vi "UnconnectedTest.vi"() -> ()   [LabVIEW 2013]
panel:
  out "x-y":u32
  in  "Y Center / mm":dbl format="%#_13g"
  in  "X Center / mm":dbl format="%#_13g"
  out "Time":dbl
  in  "Precision":i32
  in  "Radius / mm":dbl format="%#_13g"
  in  "Shape":enum16{"Self-defined", "Circle"}(ring)=enum."Circle"
  out "x resolution":dbl
  out "y resolution":dbl
  out "X":i32
  out "Y":i32
  out "Case":i16
  out "XY Graph":cluster{dbl[], dbl[]}(graph)
  in  "Polygon Point":dbl[][](array[numeric])
  in  "Size input solution":enum16{"Dynamic Size", "Fixed Size"}(ring)=enum."Fixed Size"
  in  "Y move Maximum / mm":dbl
  in  "X move Maximum / mm":dbl
  in  "Y step / mm":dbl
  in  "X step / mm":dbl
  in  "Initial YPos / mm":dbl
  in  "Initial XPos / mm":dbl
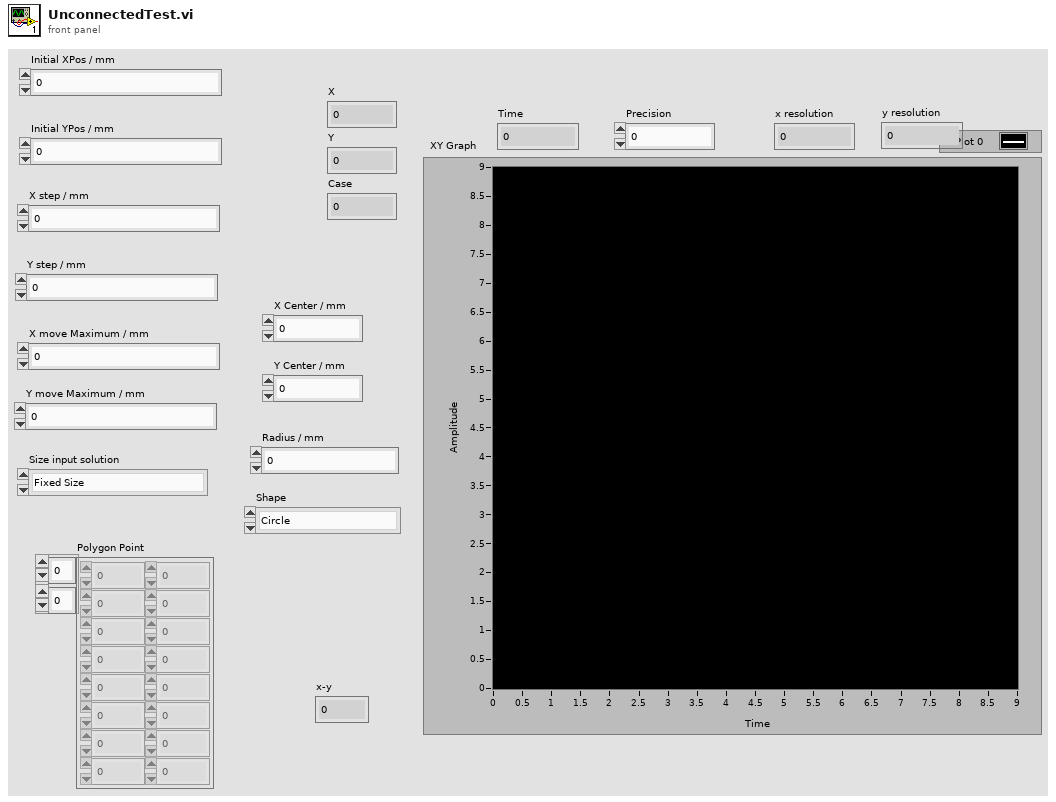
[diagram p1: front panel]
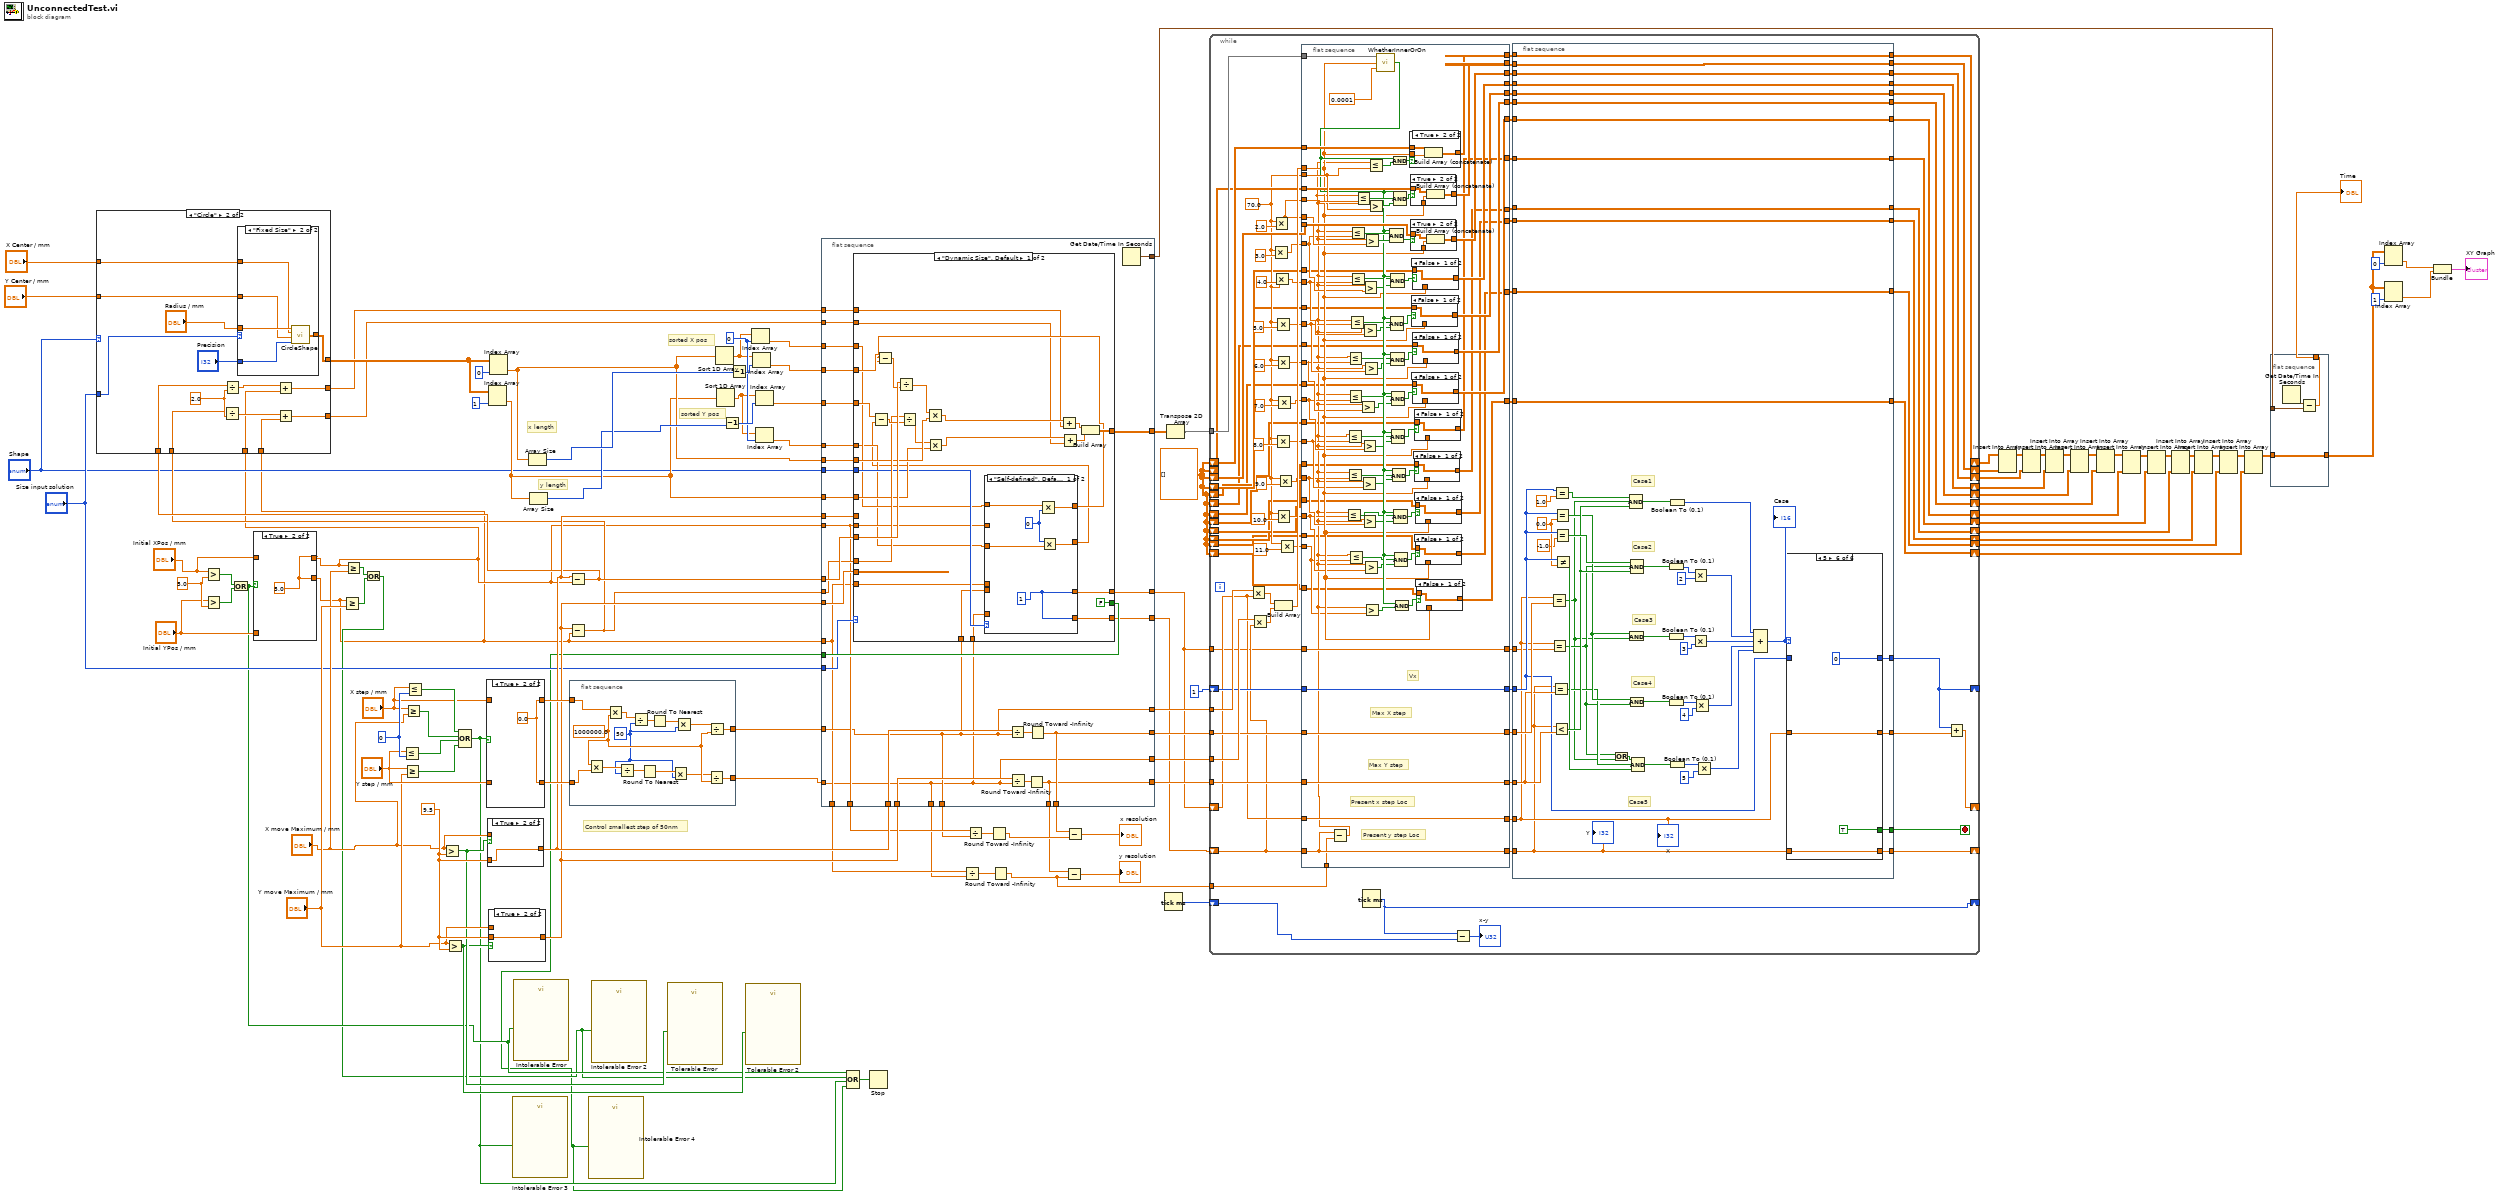
[diagram p0: block diagram]
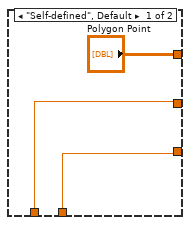
[diagram p2: hidden frame]
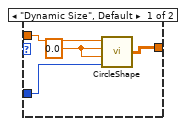
[diagram p3: hidden frame]
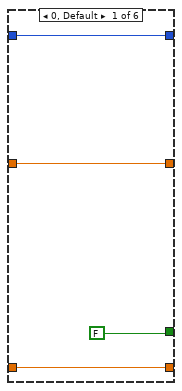
[diagram p4: hidden frame]
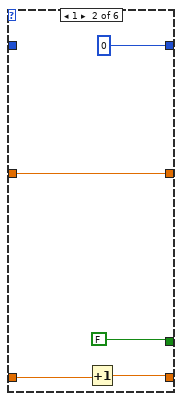
[diagram p5: hidden frame]
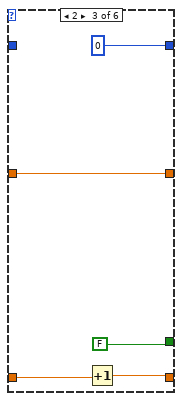
[diagram p6: hidden frame]
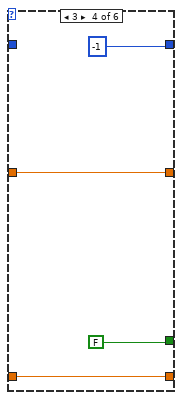
[diagram p7: hidden frame]
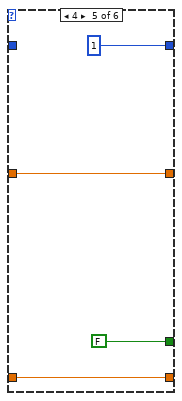
[diagram p8: hidden frame]
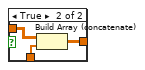
[diagram p9: hidden frame]
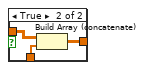
[diagram p10: hidden frame]
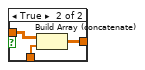
[diagram p11: hidden frame]
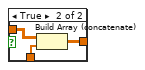
[diagram p12: hidden frame]
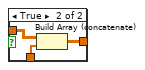
[diagram p13: hidden frame]
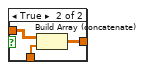
[diagram p14: hidden frame]
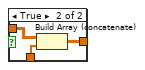
[diagram p15: hidden frame]
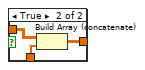
[diagram p16: hidden frame]
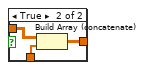
[diagram p17: hidden frame]
diagram:
  w57 = 0 ("index")
  w22 = dbl[][] []
  w104 = 0
  w105 = 9.5
  w110 = 5.0
  # "sorted Y pos"
  # "sorted X pos"
  # "Control smallest step of 50nm"
  # "y length"
  # "x length"
  n1 = Greater?(x="Initial XPos / mm", y=w110) -> (0:w109:bool)
  n2 = Greater?(x="Initial YPos / mm", y=w110) -> (0:w108:bool)
  n3 = Or(x=w109, y=w108) -> (x .or. y?=w64:bool)
  n4 = case shown="True" w64 {
    tunnel: "Initial XPos / mm" -> [w112 _]
    tunnel: "Initial YPos / mm" -> [w111 _]
    tunnel: [w112 w113] -> w45
    tunnel: [w111 w113] -> w44
    frame False {
    }
    frame True {
      w113 = 5.0
    }
  }
  n5 = Greater Or Equal?(x=w44, y="Y move Maximum / mm") -> (x >= y?=w92:bool)
  n6 = Greater Or Equal?(x=w45, y="X move Maximum / mm") -> (x >= y?=w93:bool)
  n7 = Or(x=w93, y=w92) -> (x .or. y?=w63:bool)
  n8 = Less Or Equal?(x="Y step / mm", y=w104) -> (x <= y?=w101:bool)
  n9 = Greater Or Equal?(x="Y step / mm", y="Y move Maximum / mm") -> (x >= y?=w100:bool)
  n10 = Greater Or Equal?(x="X step / mm", y="X move Maximum / mm") -> (x >= y?=w102:bool)
  n11 = Less Or Equal?(x="X step / mm", y=w104) -> (x <= y?=w103:bool)
  n12 = Greater?(x="X move Maximum / mm", y=w105) -> (0:w91:bool)
  n13 = Greater?(x="Y move Maximum / mm", y=w105) -> (0:w90:bool)
  n14 = Compound Arithmetic op=OR(w103, w102, w101, w100) -> (w62:bool)
  n15 = case shown="True" w62 {
    tunnel: "X step / mm" -> [w115 _]
    tunnel: "Y step / mm" -> [w114 _]
    tunnel: [w115 w116] -> w89
    tunnel: [w114 w116] -> w88
    frame False {
    }
    frame True {
      w116 = 0.0
    }
  }
  n16 = case shown="True" w91 {
    tunnel: w105 -> [_ w118]
    tunnel: "X move Maximum / mm" -> [w117 _]
    tunnel: [w117 w118] -> w77
    frame False {
    }
    frame True {
    }
  }
  n17 = case shown="True" w90 {
    tunnel: w105 -> [_ w120]
    tunnel: "Y move Maximum / mm" -> [w119 _]
    tunnel: [w119 w120] -> w76
    frame False {
    }
    frame True {
    }
  }
  n18 = call "Intolerable Error 3"("Enable"=w62) -> ()  [unwired: 9 in, 2 out]
  n19 = call "Intolerable Error"("Enable"=w64) -> ()  [unwired: 9 in, 2 out]
  n20 = Subtract(x=w77, y=w45) -> (x-y=w70:dbl)
  n21 = Subtract(x=w76, y=w44) -> (x-y=w69:dbl)
  n22 = case shown="\"Circle\"" "Shape" {
    tunnel: ["Polygon Point" w136] -> w79
    tunnel: "Size input solution" -> [_ w135]
    tunnel: w70 -> [_ w131]
    tunnel: w69 -> [_ w130]
    tunnel: w44 -> [w121 w129]
    tunnel: w45 -> [w122 w128]
    tunnel: [w122 w127] -> w68
    tunnel: [w121 w126] -> w67
    tunnel: "X Center / mm" -> [_ w125]
    tunnel: "Y Center / mm" -> [_ w124]
    frame "Self-defined", Default {
    }
    frame "Circle" {
      w134 = 2.0
      n23 = Divide(x=w130, y=w134) -> (x/y=w132:dbl)
      n24 = Divide(x=w131, y=w134) -> (x/y=w133:dbl)
      n25 = case shown="\"Fixed Size\"" w135 {
        tunnel: "Radius / mm" -> [w141 w147]
        tunnel: "Precision" -> [w140 w146]
        tunnel: [w142 w145] -> w136
        tunnel: w125 -> [_ w144]
        tunnel: w124 -> [_ w143]
        frame "Dynamic Size", Default {
          w139 = 0.0 ("X initial")
          n26 = call "CircleShape.vi"("Precision"=w140, "Y initial"=w139, "X initial"=w139, "Radius"=w141) -> ("Output Point"=w142:dbl[][])
        }
        frame "Fixed Size" {
          n27 = call "CircleShape.vi"("Precision"=w146, "Y initial"=w143, "X initial"=w144, "Radius"=w147) -> ("Output Point"=w145:dbl[][])
        }
      }
      n28 = Add(x=w133, y=w128) -> (x+y=w127:dbl)
      n29 = Add(x=w132, y=w129) -> (x+y=w126:dbl)
    }
  }
  n30 = Index Array(array=w79, index (col)=1 ("disabled index (col)")) -> (element=w47:dbl[])  [unwired: 1 in]
  n31 = Index Array(array=w79, index (col)=0 ("disabled index (col)")) -> (element=w48:dbl[])  [unwired: 1 in]
  n32 = Array Size(array=w48) -> (size(s)=w50:i32)
  n33 = Array Size(array=w47) -> (size(s)=w49:i32)
  n34 = flat-sequence {
    tunnel: w89 -> [w161]
    tunnel: w88 -> [w158]
    tunnel: [w154] -> w87
    tunnel: [w153] -> w86
    frame #0 {
      w150 = 50
      w155 = 1000000.0
      n35 = Multiply(x=w155, y=w158) -> (x*y=w157:dbl)
      n36 = Multiply(x=w161, y=w155) -> (x*y=w160:dbl)
      n37 = Divide(x=w157, y=w150) -> (x/y=w156:dbl)
      n38 = Divide(x=w160, y=w150) -> (x/y=w159:dbl)
      n39 = Round To Nearest(number=w156) -> (nearest integer value=w151:dbl)
      n40 = Round To Nearest(number=w159) -> (nearest integer value=w152:dbl)
      n41 = Multiply(x=w151, y=w150) -> (x*y=w149:dbl)
      n42 = Multiply(x=w152, y=w150) -> (x*y=w148:dbl)
      n43 = Divide(x=w149, y=w155) -> (x/y=w153:dbl)
      n44 = Divide(x=w148, y=w155) -> (x/y=w154:dbl)
    }
  }
  n45 = call "Intolerable Error 4"("Enable"=w61) -> ()  [unwired: 9 in, 2 out]
  n46 = call "Intolerable Error 2"("Enable"=w63) -> ()  [unwired: 9 in, 2 out]
  n47 = call "Tolerable Error"("Enable"=w91) -> ()  [unwired: 9 in, 2 out]
  n48 = Sort 1D Array(array=w48) -> (sorted array=w55:dbl[])
  n49 = Sort 1D Array(array=w47) -> (sorted array=w56:dbl[])
  n50 = Decrement(x=w49) -> (x-1=w58:i32)
  n51 = Decrement(x=w50) -> (x-1=w59:i32)
  n52 = call "Tolerable Error 2"("Enable"=w90) -> ()  [unwired: 9 in, 2 out]
  n53 = Index Array(array=w55, index=w57) -> (element=w54:dbl)
  n54 = Index Array(array=w55, index=w59) -> (element=w53:dbl)
  n55 = Index Array(array=w56, index=w58) -> (element=w52:dbl)
  n56 = Index Array(array=w56, index=w57) -> (element=w51:dbl)
  n57 = flat-sequence {
    tunnel: w70 -> [w184]
    tunnel: w69 -> [w183]
    tunnel: w77 -> [w190]
    tunnel: w45 -> [w167]
    tunnel: w76 -> [w189]
    tunnel: w44 -> [w163]
    tunnel: [w188] -> w61
    tunnel: w87 -> [w166]
    tunnel: w86 -> [w162]
    tunnel: [w187] -> w81
    tunnel: [w165] -> w85
    tunnel: [w164] -> w84
    tunnel: [w162] -> w83
    tunnel: [w166] -> w82
    tunnel: [w182] -> w78
    tunnel: w68 -> [w181]
    tunnel: w67 -> [w180]
    tunnel: w77 -> [w179]
    tunnel: w76 -> [w178]
    tunnel: [w177] -> w72
    tunnel: [w176] -> w73
    tunnel: "Size input solution" -> [w175]
    tunnel: w54 -> [w174]
    tunnel: w53 -> [w173]
    tunnel: w52 -> [w172]
    tunnel: w51 -> [w171]
    tunnel: w48 -> [w170]
    tunnel: w47 -> [w169]
    tunnel: "Shape" -> [w168]
    tunnel: [w167] -> w33
    tunnel: [w166] -> w32
    tunnel: [w165] -> w30
    tunnel: [w164] -> w26
    tunnel: [w163] -> w25
    tunnel: [w162] -> w24
    frame #0 {
      n58 = case shown="\"Dynamic Size\", Default" w175 {
        tunnel: w170 -> [w213 w241]
        tunnel: w169 -> [w212 w240]
        tunnel: w173 -> [w219 w256]
        tunnel: w174 -> [w198 w254]
        tunnel: w172 -> [w218 w252]
        tunnel: w171 -> [w196 w249]
        tunnel: w184 -> [w217 _]
        tunnel: w183 -> [w214 _]
        tunnel: [w199 w242] -> w187
        tunnel: w190 -> [_ w255]
        tunnel: w167 -> [w207 w253]
        tunnel: w189 -> [_ w251]
        tunnel: w163 -> [w206 w250]
        tunnel: [FALSE w243] -> w188
        tunnel: w181 -> [w191 _]
        tunnel: w180 -> [w192 _]
        tunnel: w166 -> [w205 _]
        tunnel: w162 -> [w204 _]
        tunnel: [w202 w239] -> w177
        tunnel: [w203 w239] -> w176
        tunnel: w168 -> [w208 _]
        frame "Dynamic Size", Default {
          n59 = case shown="\"Self-defined\", Default" w208 {
            tunnel: w207 -> [_ w236]
            tunnel: w206 -> [_ w235]
            tunnel: w205 -> [_ w234]
            tunnel: w204 -> [_ w233]
            tunnel: [w225 w232] -> w203
            tunnel: [w225 w231] -> w202
            tunnel: w198 -> [w224 w230]
            tunnel: [w221 w229] -> w197
            tunnel: w196 -> [w223 w228]
            tunnel: [w220 w226] -> w195
            frame "Self-defined", Default {
              w222 = 0
              w225 = 1
              n60 = Multiply(x=w224, y=w222) -> (x*y=w221:dbl)
              n61 = Multiply(x=w222, y=w223) -> (x*y=w220:dbl)
            }
            frame "Circle" {
              w227 = 1.0
              n62 = Divide(x=w235, y=w233) -> (x/y=w237:dbl)
              n63 = Divide(x=w236, y=w234) -> (x/y=w238:dbl)
              n64 = Multiply(x=w230, y=w227) -> (x*y=w229:dbl)
              n65 = Multiply(x=w227, y=w228) -> (x*y=w226:dbl)
              n66 = Round Toward -Infinity(1:w238) -> (0:w232:dbl)
              n67 = Round Toward -Infinity(1:w237) -> (0:w231:dbl)
            }
          }
          n68 = Subtract(x=w218, y=w195) -> (x-y=w215:dbl)
          n69 = Subtract(x=w219, y=w197) -> (x-y=w216:dbl)
          n70 = Divide(x=w217, y=w216) -> (x/y=w194:dbl)
          n71 = Divide(x=w214, y=w215) -> (x/y=w193:dbl)
          n72 = Multiply(x=w194, y=w213) -> (x*y=w210:dbl[])
          n73 = Multiply(x=w193, y=w212) -> (x*y=w209:dbl[])
          n74 = Add(x=w210, y=w191) -> (x+y=w201:dbl[])
          n75 = Add(x=w209, y=w192) -> (x+y=w200:dbl[])
          n76 = Build Array(w201, w200) -> (w199:dbl[][])
        }
        frame "Fixed Size" {
          w239 = 1
          n77 = Greater?(x=w256, y=w255) -> (0:w247:bool)
          n78 = Less?(x=w254, y=w253) -> (x < y?=w248:bool)
          n79 = Greater?(x=w252, y=w251) -> (0:w246:bool)
          n80 = Less?(x=w249, y=w250) -> (x < y?=w245:bool)
          n81 = Compound Arithmetic op=OR(w248, w247, w246, w245) -> (w244:bool)
          n82 = case shown="True" w244 {
            tunnel: [FALSE TRUE] -> w243
            frame False {
            }
            frame True {
            }
          }
          n83 = Build Array(w241, w240) -> (w242:dbl[][])
        }
      }
      n84 = Divide(x=w179, y=w166) -> (x/y=w186:dbl)
      n85 = Divide(x=w178, y=w162) -> (x/y=w185:dbl)
      n86 = Round Toward -Infinity(1:w185) -> (0:w164:dbl)
      n87 = Round Toward -Infinity(1:w186) -> (0:w165:dbl)
      n88 = Get Date/Time In Seconds() -> (seconds since 1Jan1904=w182:timestamp)
    }
  }
  n89 = Compound Arithmetic op=OR(w64, w63, w62, w61) -> (w60:bool)
  n90 = Stop(stop? (T)=w60) -> ()
  n91 = Divide(x=w25, y=w24) -> (x/y=w27:dbl)
  n92 = Divide(x=w33, y=w32) -> (x/y=w34:dbl)
  n93 = Round Toward -Infinity(1:w34) -> (0:w29:dbl)
  n94 = Round Toward -Infinity(1:w27) -> (0:w23:dbl)
  n95 = Subtract(x=w26, y=w23) -> (x-y=→"y resolution":dbl)
  n96 = Subtract(x=w30, y=w29) -> (x-y=→"x resolution":dbl)
  n97 = Tick Count (ms)() -> (millisecond timer value=w43:u32)
  n98 = Transpose 2D Array(2D array=w81) -> (transposed array=w80:dbl[][])
  n99 = while {
    tunnel: w85 -> [w331]
    tunnel: w84 -> [w329]
    tunnel: w80 -> [w337]
    tunnel: w83 -> [w341]
    tunnel: w82 -> [w342]
    shift-right: [w322] -> _
    shift-left: 1 -> [w333]
    shift-right: [w321] -> _
    shift-left: w73 -> [w327]
    shift-right: [w320] -> _
    shift-left: w72 -> [w325]
    shift-right: [w319] -> w36
    shift-left: w22 -> [w336]
    tunnel: w73 -> [w317]
    shift-right: [w315] -> _
    shift-left: w43 -> [w316]
    shift-right: [w311] -> w35
    shift-left: w22 -> [w310]
    tunnel: w23 -> [w309]
    shift-right: [w304] -> w16
    shift-left: w22 -> [w306]
    shift-right: [w283] -> w15
    shift-left: w22 -> [w285]
    shift-right: [w280] -> w14
    shift-left: w22 -> [w282]
    shift-right: [w277] -> w13
    shift-left: w22 -> [w279]
    shift-right: [w274] -> w12
    shift-left: w22 -> [w276]
    shift-right: [w271] -> w10
    shift-left: w22 -> [w273]
    shift-right: [w268] -> w8
    shift-left: w22 -> [w270]
    shift-right: [w265] -> w7
    shift-left: w22 -> [w267]
    shift-right: [w262] -> w5
    shift-left: w22 -> [w264]
    shift-right: [w259] -> w2
    shift-left: w22 -> [w261]
    stop <- w324 stop-if-true
    w293 = 70.0
    n100 = Multiply(x=w342, y=w327) -> (x*y=w340:dbl)
    n101 = Multiply(x=w341, y=w325) -> (x*y=w339:dbl)
    n102 = Multiply(x=w293, y=3.0) -> (x*y=w303:dbl)
    n103 = Multiply(x=w293, y=2.0) -> (x*y=w308:dbl)
    n104 = Multiply(x=w293, y=4.0) -> (x*y=w299:dbl)
    n105 = Multiply(x=w293, y=5.0) -> (x*y=w292:dbl)
    n106 = Multiply(x=w293, y=8.0) -> (x*y=w289:dbl)
    n107 = Multiply(x=w293, y=6.0) -> (x*y=w291:dbl)
    n108 = Multiply(x=w293, y=10.0) -> (x*y=w287:dbl)
    n109 = Build Array(w340, w339) -> (w338:dbl[])
    n110 = Multiply(x=w293, y=7.0) -> (x*y=w290:dbl)
    n111 = Multiply(x=w293, y=9.0) -> (x*y=w288:dbl)
    n112 = Multiply(x=w293, y=11.0) -> (x*y=w286:dbl)
    n113 = flat-sequence {
      tunnel: w338 -> [w451]
      tunnel: w337 -> [w498]
      tunnel: w336 -> [w488]
      tunnel: [w503] -> w335
      tunnel: [w502] -> w334
      tunnel: w333 -> [w502]
      tunnel: [w501] -> w332
      tunnel: w331 -> [w501]
      tunnel: [w500] -> w330
      tunnel: w329 -> [w500]
      tunnel: [w499] -> w328
      tunnel: w327 -> [w499]
      tunnel: [w485] -> w326
      tunnel: w325 -> [w485]
      tunnel: [w496] -> w318
      tunnel: w317 -> [w496]
      tunnel: w293 -> [w489]
      tunnel: w308 -> [w490]
      tunnel: [w487] -> w312
      tunnel: w310 -> [w486]
      tunnel: w309 -> [w484]
      tunnel: w308 -> [w478]
      tunnel: w306 -> [w480]
      tunnel: [w479] -> w305
      tunnel: w303 -> [w450]
      tunnel: w299 -> [w448]
      tunnel: w292 -> [w447]
      tunnel: w291 -> [w446]
      tunnel: w290 -> [w445]
      tunnel: w289 -> [w444]
      tunnel: w288 -> [w443]
      tunnel: w287 -> [w442]
      tunnel: w286 -> [w440]
      tunnel: w285 -> [w439]
      tunnel: [w438] -> w284
      tunnel: w282 -> [w437]
      tunnel: [w436] -> w281
      tunnel: w279 -> [w435]
      tunnel: [w434] -> w278
      tunnel: w276 -> [w433]
      tunnel: [w432] -> w275
      tunnel: w273 -> [w431]
      tunnel: [w430] -> w272
      tunnel: w270 -> [w429]
      tunnel: [w428] -> w269
      tunnel: w267 -> [w427]
      tunnel: [w426] -> w266
      tunnel: w264 -> [w425]
      tunnel: [w424] -> w263
      tunnel: w261 -> [w423]
      tunnel: [w422] -> w260
      frame #0 {
        # "Max X step"
        # "Max Y step"
        # "Present y step Loc"
        # "Present x step Loc"
        # "Vx"
        n114 = Subtract(x=w485, y=w484) -> (x-y=w441:dbl)
        n115 = Less Or Equal?(x=w441, y=w442) -> (x <= y?=w455:bool)
        n116 = Less Or Equal?(x=w441, y=w444) -> (x <= y?=w459:bool)
        n117 = Less Or Equal?(x=w441, y=w443) -> (x <= y?=w457:bool)
        n118 = Less Or Equal?(x=w441, y=w446) -> (x <= y?=w463:bool)
        n119 = Less Or Equal?(x=w441, y=w445) -> (x <= y?=w461:bool)
        n120 = Less Or Equal?(x=w441, y=w440) -> (x <= y?=w453:bool)
        n121 = Less Or Equal?(x=w441, y=w447) -> (x <= y?=w465:bool)
        n122 = Less Or Equal?(x=w441, y=w450) -> (x <= y?=w482:bool)
        n123 = Less Or Equal?(x=w441, y=w448) -> (x <= y?=w467:bool)
        n124 = Less Or Equal?(x=w441, y=w490) -> (x <= y?=w492:bool)
        n125 = Greater?(x=w441, y=w446) -> (0:w460:bool)
        n126 = Greater?(x=w441, y=w444) -> (0:w456:bool)
        n127 = Greater?(x=w441, y=w445) -> (0:w458:bool)
        n128 = Greater?(x=w441, y=w443) -> (0:w454:bool)
        n129 = Greater?(x=w441, y=w448) -> (0:w464:bool)
        n130 = Greater?(x=w441, y=w450) -> (0:w466:bool)
        n131 = Greater?(x=w441, y=w447) -> (0:w462:bool)
        n132 = Greater?(x=w441, y=w442) -> (0:w452:bool)
        n133 = Greater?(x=w441, y=w478) -> (0:w481:bool)
        n134 = Greater?(x=w441, y=w440) -> (0:w449:bool)
        n135 = Less Or Equal?(x=w441, y=w489) -> (x <= y?=w494:bool)
        n136 = Greater?(x=w441, y=w489) -> (0:w491:bool)
        n137 = call "WhetherInnerOrOn.vi"("Error permitted"=0.0001, "JudgePoint"=w451, "InputPolygon"=w498) -> ("Point on or inside?"=w468:bool)
        n138 = Compound Arithmetic op=AND(w468, w482, w481) -> (w483:bool)
        n139 = Compound Arithmetic op=AND(w468, w465, w464) -> (w476:bool)
        n140 = And(x=w468, y=w494) -> (x .and. y?=w495:bool)
        n141 = Compound Arithmetic op=AND(w468, w467, w466) -> (w477:bool)
        n142 = Compound Arithmetic op=AND(w468, w463, w462) -> (w475:bool)
        n143 = Compound Arithmetic op=AND(w468, w461, w460) -> (w474:bool)
        n144 = Compound Arithmetic op=AND(w468, w459, w458) -> (w473:bool)
        n145 = Compound Arithmetic op=AND(w468, w457, w456) -> (w472:bool)
        n146 = Compound Arithmetic op=AND(w468, w492, w491) -> (w493:bool)
        n147 = Compound Arithmetic op=AND(w468, w455, w454) -> (w471:bool)
        n148 = Compound Arithmetic op=AND(w468, w453, w452) -> (w470:bool)
        n149 = Compound Arithmetic op=AND(w468, w449) -> (w469:bool)
        n150 = case shown="True" w495 {
          tunnel: w488 -> [w548 w551]
          tunnel: w451 -> [_ w550]
          tunnel: [w548 w549] -> w503
          frame False {
          }
          frame True {
            n151 = Build Array (concatenate)(w551, w550) -> (w549:dbl[][])
          }
        }
        n152 = case shown="True" w493 {
          tunnel: w451 -> [_ w547]
          tunnel: w486 -> [w544 w546]
          tunnel: [w544 w545] -> w487
          frame False {
          }
          frame True {
            n153 = Build Array (concatenate)(w546, w547) -> (w545:dbl[][])
          }
        }
        n154 = case shown="True" w483 {
          tunnel: w451 -> [_ w543]
          tunnel: w480 -> [w540 w542]
          tunnel: [w540 w541] -> w479
          frame False {
          }
          frame True {
            n155 = Build Array (concatenate)(w542, w543) -> (w541:dbl[][])
          }
        }
        n156 = case shown="False" w476 {
          tunnel: w451 -> [_ w507]
          tunnel: [w504 w506] -> w436
          tunnel: w437 -> [w504 w505]
          frame False {
          }
          frame True {
            n157 = Build Array (concatenate)(w505, w507) -> (w506:dbl[][])
          }
        }
        n158 = case shown="False" w477 {
          tunnel: w451 -> [_ w539]
          tunnel: [w536 w538] -> w438
          tunnel: w439 -> [w536 w537]
          frame False {
          }
          frame True {
            n159 = Build Array (concatenate)(w537, w539) -> (w538:dbl[][])
          }
        }
        n160 = case shown="False" w474 {
          tunnel: w451 -> [_ w531]
          tunnel: [w528 w530] -> w432
          tunnel: w433 -> [w528 w529]
          frame False {
          }
          frame True {
            n161 = Build Array (concatenate)(w529, w531) -> (w530:dbl[][])
          }
        }
        n162 = case shown="False" w475 {
          tunnel: w451 -> [_ w535]
          tunnel: [w532 w534] -> w434
          tunnel: w435 -> [w532 w533]
          frame False {
          }
          frame True {
            n163 = Build Array (concatenate)(w533, w535) -> (w534:dbl[][])
          }
        }
        n164 = case shown="False" w472 {
          tunnel: w451 -> [_ w523]
          tunnel: [w520 w522] -> w428
          tunnel: w429 -> [w520 w521]
          frame False {
          }
          frame True {
            n165 = Build Array (concatenate)(w521, w523) -> (w522:dbl[][])
          }
        }
        n166 = case shown="False" w473 {
          tunnel: w451 -> [_ w527]
          tunnel: [w524 w526] -> w430
          tunnel: w431 -> [w524 w525]
          frame False {
          }
          frame True {
            n167 = Build Array (concatenate)(w525, w527) -> (w526:dbl[][])
          }
        }
        n168 = case shown="False" w471 {
          tunnel: w451 -> [_ w519]
          tunnel: [w516 w518] -> w426
          tunnel: w427 -> [w516 w517]
          frame False {
          }
          frame True {
            n169 = Build Array (concatenate)(w517, w519) -> (w518:dbl[][])
          }
        }
        n170 = case shown="False" w470 {
          tunnel: w451 -> [_ w515]
          tunnel: [w512 w514] -> w424
          tunnel: w425 -> [w512 w513]
          frame False {
          }
          frame True {
            n171 = Build Array (concatenate)(w513, w515) -> (w514:dbl[][])
          }
        }
        n172 = case shown="False" w469 {
          tunnel: w451 -> [_ w511]
          tunnel: [w508 w510] -> w422
          tunnel: w423 -> [w508 w509]
          frame False {
          }
          frame True {
            n173 = Build Array (concatenate)(w509, w511) -> (w510:dbl[][])
          }
        }
      }
    }
    n174 = Tick Count (ms)() -> (millisecond timer value=w315:u32)
    n175 = Subtract(x=w315, y=w316) -> (x-y=→"x-y":u32)
    n176 = flat-sequence {
      tunnel: w335 -> [w358]
      tunnel: w334 -> [w365]
      tunnel: w332 -> [w395]
      tunnel: w330 -> [w393]
      tunnel: w328 -> [w364]
      tunnel: w326 -> [w363]
      tunnel: [w362] -> w324
      tunnel: [w361] -> w323
      tunnel: [w360] -> w322
      tunnel: [w359] -> w320
      tunnel: [w358] -> w319
      tunnel: w318 -> [w357]
      tunnel: w312 -> [w353]
      tunnel: [w353] -> w311
      tunnel: w305 -> [w352]
      tunnel: [w352] -> w304
      tunnel: [w351] -> w283
      tunnel: w284 -> [w351]
      tunnel: w281 -> [w350]
      tunnel: [w350] -> w280
      tunnel: w278 -> [w349]
      tunnel: [w349] -> w277
      tunnel: w275 -> [w348]
      tunnel: [w348] -> w274
      tunnel: w272 -> [w347]
      tunnel: [w347] -> w271
      tunnel: w269 -> [w346]
      tunnel: [w346] -> w268
      tunnel: w266 -> [w345]
      tunnel: [w345] -> w265
      tunnel: w263 -> [w344]
      tunnel: [w344] -> w262
      tunnel: w260 -> [w343]
      tunnel: [w343] -> w259
      frame #0 {
        w355 = 0.0
        # "Case5"
        # "Case4"
        # "Case3"
        # "Case2"
        # "Case1"
        n177 = Equal?(x=w364, y=w395) -> (x = y?=w385:bool)
        n178 = Equal?(x=w364, y=w357) -> (x = y?=w386:bool)
        n179 = Equal?(x=w363, y=w393) -> (x = y?=w387:bool)
        n180 = Less?(x=w363, y=w393) -> (x < y?=w391:bool)
        n181 = Equal?(x=w365, y=1.0) -> (x = y?=w394:bool)
        n182 = Equal?(x=w365, y=w355) -> (x = y?=w390:bool)
        n183 = Equal?(x=w365, y=-1.0) -> (x = y?=w392:bool)
        n184 = Not Equal?(x=w365, y=w355) -> (x != y?=w388:bool)
        n185 = Or(x=w386, y=w385) -> (x .or. y?=w389:bool)
        n186 = Compound Arithmetic op=AND(w394, w385, w391) -> (w384:bool)
        n187 = Compound Arithmetic op=AND(w390, w385) -> (w382:bool)
        n188 = Compound Arithmetic op=AND(w392, w386, w391) -> (w383:bool)
        n189 = Compound Arithmetic op=AND(w390, w386) -> (w381:bool)
        n190 = Compound Arithmetic op=AND(w389, w387, w388) -> (w380:bool)
        n191 = Boolean To (0,1)(Boolean=w382) -> (0, 1=w375:i16)
        n192 = Boolean To (0,1)(Boolean=w381) -> (0, 1=w373:i16)
        n193 = Boolean To (0,1)(Boolean=w383) -> (0, 1=w377:i16)
        n194 = Boolean To (0,1)(Boolean=w384) -> (0, 1=w378:i16)
        n195 = Boolean To (0,1)(Boolean=w380) -> (0, 1=w371:i16)
        n196 = Multiply(x=w377, y=i16 2) -> (x*y=w369:i16)
        n197 = Multiply(x=w375, y=i16 3) -> (x*y=w368:i16)
        n198 = Multiply(x=w373, y=i16 4) -> (x*y=w367:i16)
        n199 = Multiply(x=w371, y=i16 5) -> (x*y=w366:i16)
        n200 = Compound Arithmetic op=ADD(w378, w369, w368, w367, w366) -> (w379:i16)
        "Case" <- w379
        n201 = case shown="5" w379 {
          tunnel: w365 -> [w399 _ _ _ _ _]
          tunnel: w364 -> [w398 w401 w406 w412 w416 w421]
          tunnel: w363 -> [w397 w403 w408 w411 w415 w420]
          tunnel: [w399 0 0 -1 1 0] -> w360
          tunnel: [w398 w401 w406 w412 w416 w421] -> w361
          tunnel: [w397 w402 w407 w411 w415 w420] -> w359
          tunnel: [FALSE FALSE FALSE FALSE FALSE TRUE] -> w362
          frame 0, Default {
          }
          frame 1 {
            n202 = Increment(x=w403) -> (x+1=w402:dbl)
          }
          frame 2 {
            n203 = Increment(x=w408) -> (x+1=w407:dbl)
          }
          frame 3 {
          }
          frame 4 {
          }
          frame 5 {
          }
        }
        "X" <- w364
        "Y" <- w363
      }
    }
    n204 = Add(x=w322, y=w323) -> (x+y=w321:dbl)
  }
  n205 = Insert Into Array(array=w36, new element=w35) -> (w21:dbl[][])  [unwired: 2 in]
  n206 = Insert Into Array(array=w21, new element=w16) -> (w20:dbl[][])  [unwired: 2 in]
  n207 = Insert Into Array(array=w20, new element=w15) -> (w19:dbl[][])  [unwired: 2 in]
  n208 = Insert Into Array(array=w19, new element=w14) -> (w18:dbl[][])  [unwired: 2 in]
  n209 = Insert Into Array(array=w18, new element=w13) -> (w17:dbl[][])  [unwired: 2 in]
  n210 = Insert Into Array(array=w17, new element=w12) -> (w11:dbl[][])  [unwired: 2 in]
  n211 = Insert Into Array(array=w11, new element=w10) -> (w9:dbl[][])  [unwired: 2 in]
  n212 = Insert Into Array(array=w9, new element=w8) -> (w6:dbl[][])  [unwired: 2 in]
  n213 = Insert Into Array(array=w6, new element=w7) -> (w4:dbl[][])  [unwired: 2 in]
  n214 = Insert Into Array(array=w4, new element=w5) -> (w3:dbl[][])  [unwired: 2 in]
  n215 = Insert Into Array(array=w3, new element=w2) -> (w1:dbl[][])  [unwired: 2 in]
  n216 = flat-sequence {
    tunnel: [w555] -> w37
    tunnel: w1 -> [w555]
    tunnel: w78 -> [w553]
    tunnel: [w552] -> w74
    frame #0 {
      n217 = Get Date/Time In Seconds() -> (seconds since 1Jan1904=w554:timestamp)
      n218 = Subtract(x=w554, y=w553) -> (x-y=w552:dbl)
    }
  }
  n219 = Index Array(array=w37, index (col)=0 ("disabled index (col)")) -> (element=w40:dbl[])  [unwired: 1 in]
  n220 = Index Array(array=w37, index (col)=1 ("disabled index (col)")) -> (element=w41:dbl[])  [unwired: 1 in]
  n221 = Bundle(w40, w41) -> (→"XY Graph":cluster{dbl[], dbl[]})  [unwired: 1 in]
  "Time" <- w74
